vi "exercice8-3.vi"() -> ()   [LabVIEW 2013]
uses:
  <vilib>/DAQmx/read.llb/DAQmx Read (Analog Wfm 1Chan 1Samp).vi
  <vilib>/Waveform/WDTFileIO.llb/ Write Waveforms to File (1D).vi
  <vilib>/DAQmx/miscellaneous.llb/DAQmx Fill In Error Info.vi
panel:
  in  "Frequence Echantillonage":dbl
  in  "Nb echantillons":dbl
  in  "Nom de tâche DAQmx":refnum<k21>
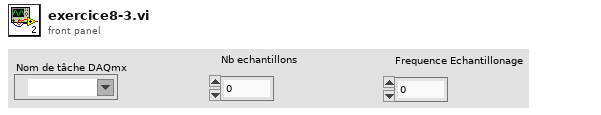
[diagram p1: front panel]
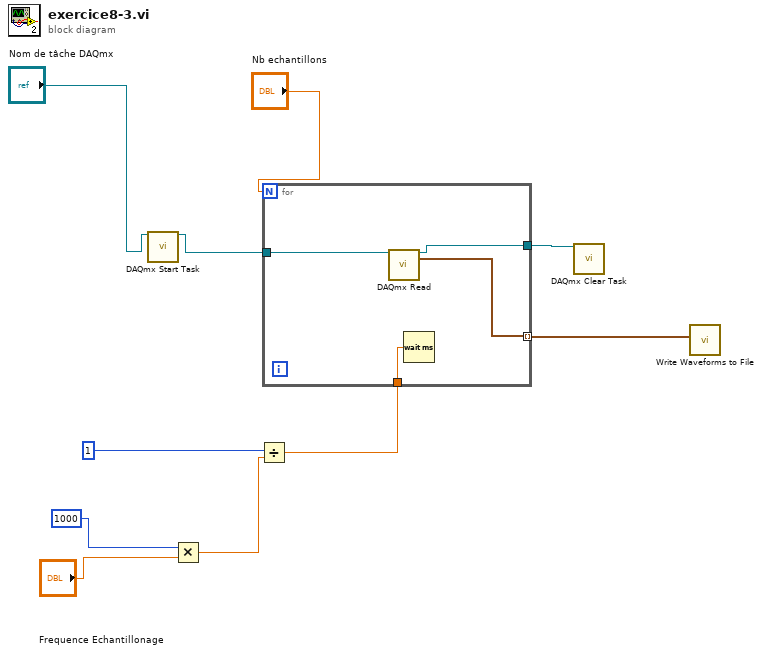
[diagram p0: block diagram]
diagram:
  n1 = call <vilib>:"DAQmx Start Task.vi"("task/channels in"="Nom de tâche DAQmx") -> ("task out"=w9:refnum<k21>)  [unwired: 13 in, 1 out]
  n2 = Multiply(x=1000, y="Frequence Echantillonage") -> (x*y=w4:dbl)
  n3 = Divide(x=1, y=w4) -> (x/y=w2:dbl)
  n4 = for {
    N: "Nb echantillons" -> [_]
    tunnel: w9 -> [w14]
    tunnel: [w13] -> w8
    tunnel: w2 -> [w12]
    tunnel: [w11] -> w1 mode=indexing
    n5 = call-poly <vilib>:"DAQmx Read.vi"("task/channels in"=w14) -> ("task out"=w13:refnum<k21>, "data"=w11:waveform(dbl))  [unwired: 12 in, 1 out]
    n6 = Wait (ms)(milliseconds to wait=w12) -> ()  [unwired: 1 out]
  }
  n7 = call <vilib>:"DAQmx Clear Task.vi"("task in"=w8) -> ()  [unwired: 14 in, 1 out]
  n8 = call-poly <vilib>:"Write Waveforms to File.vi"("waveform array"=w1) -> ()  [unwired: 9 in, 2 out]
